vi "Read Connection Event.vi"(8 "error in (no error)":errorcluster, 11 "Connection in":refnum<class "Connection.lvclass">) -> (0 "error out":errorcluster, 2 "connection event":refnum<user-event>, 3 "Connection out":refnum<class "Connection.lvclass">)   [LabVIEW 2013, in "MQTT_Connection.lvlib" / "Connection.lvclass"]
uses:
  Connection.lvclass
  connection event -- cluster.ctl
  Connection.lvclass/Connection.ctl
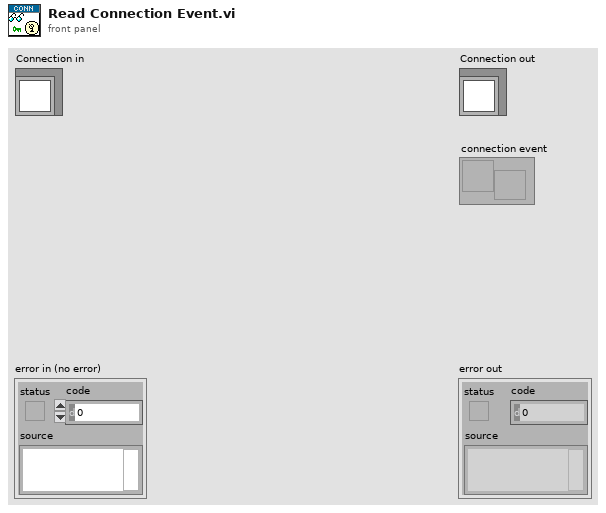
[diagram p1: front panel]
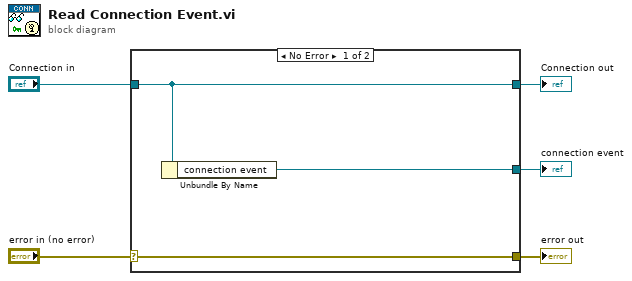
[diagram p0: block diagram]
diagram:
  n1 = case shown="No Error" "error in (no error)" {
    selector: "error in (no error)" -> [w8 w9]
    tunnel: [w8 w9] -> w4
    tunnel: [w7 w10] -> w2
    tunnel: "Connection in" -> [w7 w10]
    tunnel: [w6 _] -> w1
    frame No Error {
      n2 = Unbundle By Name(w7) -> ("connection event"=w6:refnum<user-event>)
    }
    frame Error {
    }
  }
  "error out" <- w4
  "Connection out" <- w2
  "connection event" <- w1
